vi "NestedCluster.vi"() -> ()   [LabVIEW 2014]
doc: "This example shows a simple Producer Consumer implementation on the RasPi\ntarget combined with nested data structures. Enter Command to be sent on the String control. By pressing the Send button, command is sent from Producer loop and is processed on the Consumer loop. \n\nSend:\nmultiply: will multiply values from the nested cluster by itself and display result on Cluster Indicator\nincrement: will increment values from the nested cluster by itself and display result on Cluster Indicator\nstop: will quit both parallel loops and stop the VI execution"
panel:
  out "Cluster Indicator":T1
  in  "Cluster Control":T1={"Numeric"=1.0, "Numeric 2"=3, "Numeric 3"=5.0, "Nested Cluster"={"Numeric 4"=2.0, "Numeric 5"=4, "Numeric 6"=6.0}, "Command"=""} caption="x"
  in  "Send":bool
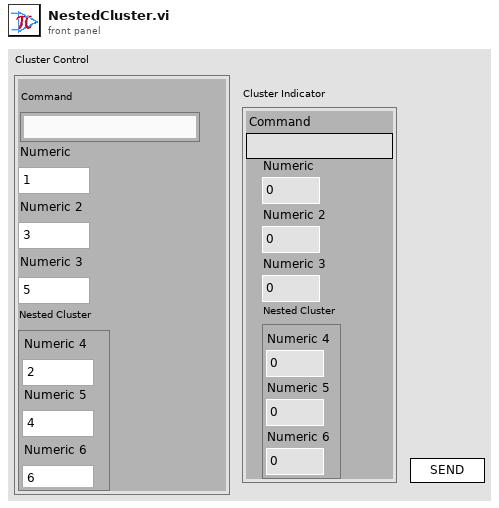
[diagram p1: front panel]
types:
  T1 = cluster{"Numeric":dbl, "Numeric 2":i32, "Numeric 3":dbl, "Nested Cluster":cluster{"Numeric 4":dbl, "Numeric 5":i32, "Numeric 6":dbl}, "Command":string}
  T2 = cluster{"Numeric 4":dbl, "Numeric 5":i32, "Numeric 6":dbl}
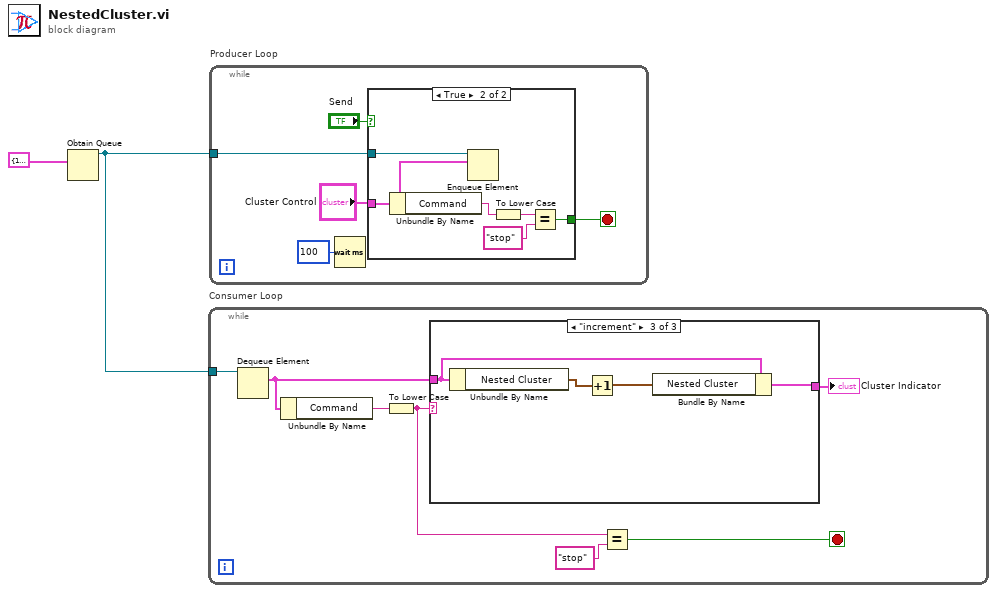
[diagram p0: block diagram]
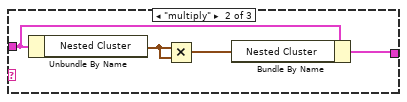
[diagram p3: hidden frame]
diagram:
  n1 = Obtain Queue(element data type=T1 {"Numeric"=1.0, "Numeric 2"=3, "Numeric 3"=5.0, "Nested Cluster"={"Numeric 4"=2.0, "Numeric 5"=4, "Numeric 6"=6.0}, "Command"=""} ("Cluster Control")) -> (queue out=w2:refnum<queue>)  [unwired: 4 in, 2 out]
  n2 = while "Consumer Loop" {
    tunnel: w2 -> [w9]
    stop <- w7 stop-if-true
    n3 = Dequeue Element(queue=w9) -> (element=w5:T1)  [unwired: 2 in, 3 out]
    n4 = Unbundle By Name(w5) -> ("Command"=w6:string)
    n5 = To Lower Case(string=w6) -> (all lower case string=w4:string)
    n6 = case shown="\"increment\"" w4 {
      tunnel: w5 -> [w10 w12 w16]
      tunnel: [w10 w11 w15] -> w3
      frame "Anything", Default {
      }
      frame "multiply" {
        n7 = Unbundle By Name(w12) -> ("Nested Cluster"=w14:T2)
        n8 = Multiply(x=w14, y=w14) -> (x*y=w13:T2)
        n9 = Bundle By Name(cluster=w12, "Nested Cluster"=w13) -> (w11:T1)
      }
      frame "increment" {
        n10 = Unbundle By Name(w16) -> ("Nested Cluster"=w18:T2)
        n11 = Increment(x=w18) -> (x+1=w17:T2)
        n12 = Bundle By Name(cluster=w16, "Nested Cluster"=w17) -> (w15:T1)
      }
    }
    "Cluster Indicator" <- w3
    n13 = Equal?(x=w4, y="stop") -> (x = y?=w7:bool)
  }
  n14 = while "Producer Loop" {
    tunnel: w2 -> [w21]
    stop <- w20 stop-if-true
    n15 = Wait (ms)(milliseconds to wait=u32 100) -> ()  [unwired: 1 out]
    n16 = case shown="True" "Send" {
      tunnel: w21 -> [_ w29]
      tunnel: "Cluster Control" -> [_ w25]
      tunnel: [_ w26] -> w20
      frame False {
      }
      frame True {
        n17 = Unbundle By Name(w25) -> ("Command"=w24:string)
        n18 = Enqueue Element(queue=w29, element=w25) -> ()  [unwired: 2 in, 3 out]
        n19 = To Lower Case(string=w24) -> (all lower case string=w27:string)
        n20 = Equal?(x=w27, y="stop") -> (x = y?=w26:bool)
      }
    }
  }
